vi "coor2id.vi"(4 "Square Periphery":i32[](array[numeric]), 5 "Size(um)":i32[](array[numeric])) -> (0 "Id":i32)   [LabVIEW 2016]
doc: "This Vi calculates the unique ID from the (x,y,z) coordinates, according to the grid size"
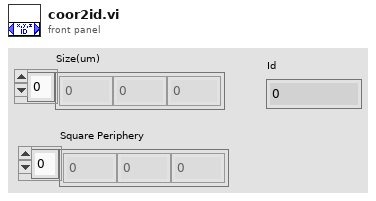
[diagram p1: front panel]
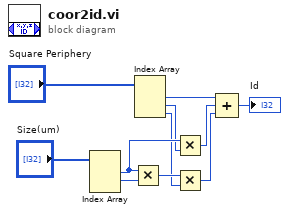
[diagram p0: block diagram]
diagram:
  n1 = Index Array(array="Size(um)") -> (element #1=w10:i32, element #2=w11:i32)  [unwired: 3 in, 1 out]
  n2 = Multiply(x=w10, y=w11) -> (x*y=w7:i32)
  n3 = Index Array(array="Square Periphery") -> (element #1=w4:i32, element #2=w5:i32, element #3=w6:i32)  [unwired: 3 in]
  n4 = Multiply(x=w10, y=w5) -> (x*y=w3:i32)
  n5 = Multiply(x=w7, y=w6) -> (x*y=w2:i32)
  n6 = Compound Arithmetic op=ADD(w4, w3, w2) -> (→"Id":i32)
